vi "Add Item To Scene.vi"(8 "error in":errorcluster, 10 "Tree Element":T1, 11 "Scene In":refnum<vi>) -> (0 "error out":errorcluster, 3 "Scene Out":refnum<vi>)   [LabVIEW 2015]
doc: "This VI adds all the items to the scene"
uses:
  <vilib>/robotics/Kinematics/Plotting/Tree Element.ctl
  <vilib>/robotics/Kinematics/Plotting/Element Type.ctl
  <vilib>/robotics/Kinematics/Plotting/Joint Type.ctl
  <vilib>/picture/3D Picture Control/Object/Create Object (name).vi
  <vilib>/Utility/AngleManip/Degrees to Radians (Scalar DBL).vi
  <vilib>/picture/3D Picture Control/NI_3D Picture Control.lvlib
  <vilib>/Utility/AngleManip/NI_AngleManipulation.lvlib
  <vilib>/robotics/Kinematics/Plotting/NI_Robotics_3DKinematics.lvlib
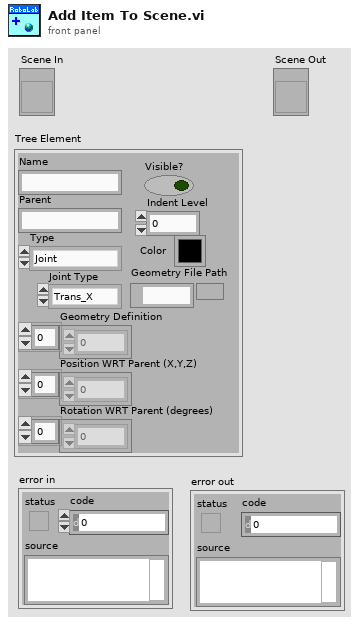
[diagram p1: front panel]
types:
  T1 = typedef "NI_Robotics_3DKinematics.lvlib/Tree Element.ctl" = cluster{"Name":string, "Parent":string, "Type":T2, "Visible?":bool, "Geometry Definition":dbl[], "Position WRT Parent (X,Y,Z)":dbl[], "Rotation WRT Parent (degrees)":dbl[], "Joint Type":T3, "Geometry File Path":path, "Indent Level":i32, "Color":u32}
  T2 = typedef "NI_Robotics_3DKinematics.lvlib/Element Type.ctl" = enum16{"Joint", "Box", "Cylinder", "Cone", "Sphere", "ASE File", "VRML File", "STL File", "Space"}
  T3 = typedef "NI_Robotics_3DKinematics.lvlib/Joint Type.ctl" = enum16{"Trans_X", "Trans_Y", "Trans_Z", "Rot_X", "Rot_Y", "Rot_Z", "None"}
  T4 = enum16{"Overall", "Per Primitive", "Per Vertex", "Binding Off"}
  T5 = cluster{"Position WRT Parent (X,Y,Z)[0]":dbl, "Position WRT Parent (X,Y,Z)[1]":dbl, "Position WRT Parent (X,Y,Z)[2]":dbl}
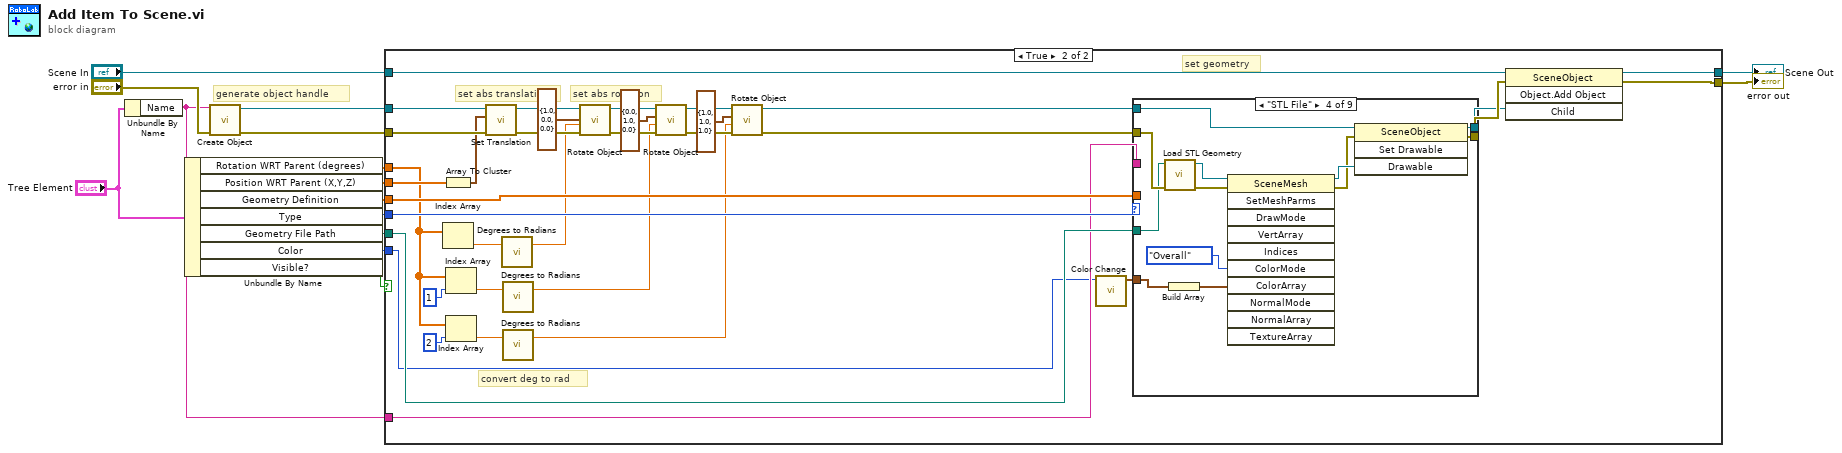
[diagram p0: block diagram]
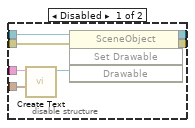
[diagram p4: hidden frame]
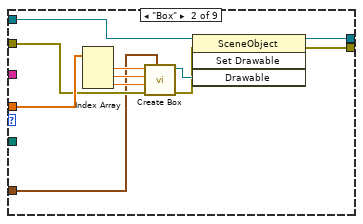
[diagram p5: hidden frame]
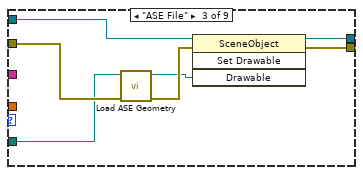
[diagram p6: hidden frame]
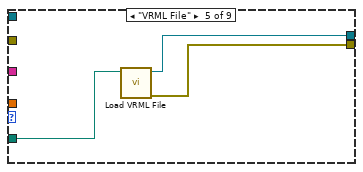
[diagram p7: hidden frame]
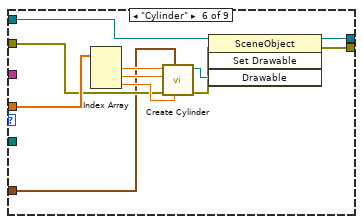
[diagram p8: hidden frame]
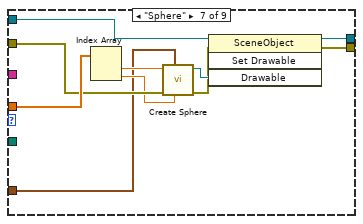
[diagram p9: hidden frame]
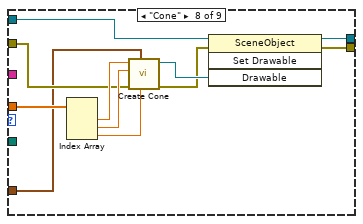
[diagram p10: hidden frame]
diagram:
  # "generate object handle"
  n1 = Unbundle By Name("Tree Element") -> ("Name"=w6:string)
  n2 = Unbundle By Name("Tree Element") -> ("Rotation WRT Parent (degrees)"=w4:dbl[], "Position WRT Parent (X,Y,Z)"=w12:dbl[], "Geometry Definition"=w10:dbl[], "Type"=w9:T2, "Geometry File Path"=w7:path, "Color"=w5:u32, "Visible?"=w1:bool)
  n3 = call-poly <vilib>:"Create Object.vi"("error in (no error)"="error in", "Name"=w6) -> ("error out"=w13:errorcluster, "Scene:New Object"=w14:refnum<vi>)  [unwired: 8 in]
  n4 = case shown="True" w1 {
    tunnel: w14 -> [_ w52]
    tunnel: w13 -> [w16 w51]
    tunnel: w12 -> [_ w50]
    tunnel: w10 -> [_ w48]
    tunnel: w9 -> [_ w46]
    tunnel: "Scene In" -> [w17 w45]
    tunnel: w7 -> [_ w44]
    tunnel: w6 -> [_ w43]
    tunnel: w5 -> [_ w32]
    tunnel: w4 -> [_ w20]
    tunnel: [w17 w19] -> w3
    tunnel: [w16 w18] -> w2
    frame False {
    }
    frame True {
      # "set abs rotation"
      # "set abs translation"
      # "set geometry"
      # "convert deg to rad"
      n5 = Array To Cluster(array=w50) -> (cluster=w39:T5)
      n6 = Index Array(array=w20) -> (element=w38:dbl)  [unwired: 1 in]
      n7 = Index Array(array=w20, index=1) -> (element=w31:dbl)
      n8 = Index Array(array=w20, index=2) -> (element=w23:dbl)
      n9 = call <vilib>:"Set Translation.vi"("error in (no error)"=w51, "Translation"=w39, "Scene Object"=w52) -> ("error out"=w41:errorcluster, "Translated Object"=w40:refnum<vi>)  [unwired: 7 out]
      n10 = call-poly <vilib>:"Degrees to Radians.vi"("angle (deg)"=w38) -> ("angle (rad)"=w37:dbl)  [unwired: 2 in]
      n11 = call-poly <vilib>:"Degrees to Radians.vi"("angle (deg)"=w31) -> ("angle (rad)"=w29:dbl)  [unwired: 2 in]
      n12 = call-poly <vilib>:"Degrees to Radians.vi"("angle (deg)"=w23) -> ("angle (rad)"=w24:dbl)  [unwired: 2 in]
      n13 = call <vilib>:"Rotate Object.vi"("error in (no error)"=w41, "Angle"=w37, "Axis"=cluster{"X":sgl, "Y":sgl, "Z":sgl} {"X"=1.0, "Y"=0.0, "Z"=0.0}, "Scene.Object In"=w40) -> ("error out"=w34:errorcluster, "Scene.Object Out"=w35:refnum<vi>)  [unwired: 6 in]
      n14 = call <vilib>:"Rotate Object.vi"("error in (no error)"=w34, "Angle"=w29, "Axis"=cluster{"X":sgl, "Y":sgl, "Z":sgl} {"X"=0.0, "Y"=1.0, "Z"=0.0}, "Scene.Object In"=w35) -> ("error out"=w27:errorcluster, "Scene.Object Out"=w28:refnum<vi>)  [unwired: 6 in]
      n15 = call <vilib>:"Rotate Object.vi"("error in (no error)"=w27, "Angle"=w24, "Axis"=cluster{"X":sgl, "Y":sgl, "Z":sgl} {"X"=1.0, "Y"=1.0, "Z"=1.0}, "Scene.Object In"=w28) -> ("error out"=w21:errorcluster, "Scene.Object Out"=w22:refnum<vi>)  [unwired: 6 in]
      n16 = call <vilib>:"Color Change.vi"("Color"=w32) -> ("RGBA"=w42:cluster{"R":sgl, "G":sgl, "B":sgl, "A":sgl})  [unwired: 1 in, 9 out]
      n17 = case shown="\"STL File\"" w46 {
        tunnel: w22 -> [w56 w78 w79 w97 _ w111 w121 w132 w134]
        tunnel: [w55 w77 w85 w96 w99 w110 w120 w131 w134] -> w47
        tunnel: w48 -> [_ w76 _ _ _ w109 w119 w130 _]
        tunnel: w21 -> [w58 w71 w84 w95 _ w104 w117 w123 w133]
        tunnel: [w54 w69 w82 w94 w98 w102 w115 w125 w133] -> w49
        tunnel: w44 -> [_ _ w81 w93 w100 _ _ _ _]
        tunnel: w43 -> [w57 _ _ _ _ _ _ _ _]
        tunnel: w42 -> [w53 w68 _ w92 _ w101 w112 w122 _]
        frame "Joint", Default {
          n18 = disable-structure shown="Enabled" {
            disable-tunnel: w58 -> [w64 w66]
            disable-tunnel: w57 -> [w63 _]
            disable-tunnel: w56 -> [w62 w67]
            disable-tunnel: [w61 w67] -> w55
            disable-tunnel: [w60 w66] -> w54
            disable-tunnel: w53 -> [w59 _]
            frame Disabled {
              n19 = call <vilib>:"Create Text.vi"("Color"=w59, "Text"=w63) -> ("New Text Refnum"=w65:refnum<vi>)  [unwired: 2 in, 7 out]
              n20 = invoke class="SceneObject" method="Set Drawable"(reference=w62, error in=w64, "Drawable"=w65) -> (reference out=w61:refnum<vi>, error out=w60:errorcluster)  [unwired: 1 in, 2 out]
            }
            frame Enabled {
            }
          }
        }
        frame "Box" {
          n21 = Index Array(array=w76) -> (element #1=w75:dbl, element #2=w74:dbl, element #3=w73:dbl)  [unwired: 3 in]
          n22 = call <vilib>:"Create Box.vi"("Color"=w68, "error in (no error)"=w71, "Length Z"=w73, "Length Y"=w74, "Length X"=w75) -> ("error out"=w70:errorcluster, "New Box Refnum"=w72:refnum<vi>)  [unwired: 5 out]
          n23 = invoke class="SceneObject" method="Set Drawable"(reference=w78, error in=w70, "Drawable"=w72) -> (reference out=w77:refnum<vi>, error out=w69:errorcluster)  [unwired: 1 in, 2 out]
        }
        frame "ASE File" {
          n24 = call <vilib>:"Load ASE Geometry.vi"("error in (no error)"=w84, "Model File"=w81) -> ("error out"=w83:errorcluster, "New Mesh Refnum"=w80:refnum<vi>)  [unwired: 2 in, 6 out]
          n25 = invoke class="SceneObject" method="Set Drawable"(reference=w79, error in=w83, "Drawable"=w80) -> (reference out=w85:refnum<vi>, error out=w82:errorcluster)  [unwired: 1 in, 2 out]
        }
        frame "STL File" {
          n26 = call <vilib>:"Load STL Geometry.vi"("error in (no error)"=w95, "Model File"=w93) -> ("error out"=w87:errorcluster, "New Mesh Refnum"=w91:refnum<vi>)  [unwired: 8 out]
          n27 = Build Array(w92) -> (w88:cluster{"R":sgl, "G":sgl, "B":sgl, "A":sgl}[])
          n28 = invoke class="SceneMesh" method="SetMeshParms"(reference=w91, error in=w87, "ColorMode"=T4."Overall" ("Color Binding Mode"), "ColorArray"=w88) -> (reference out=w90:refnum<vi>, error out=w86:errorcluster)  [unwired: 7 in, 9 out]
          n29 = invoke class="SceneObject" method="Set Drawable"(reference=w97, error in=w86, "Drawable"=w90) -> (reference out=w96:refnum<vi>, error out=w94:errorcluster)  [unwired: 1 in, 2 out]
        }
        frame "VRML File" {
          n30 = call <vilib>:"Load VRML File.vi"("Path"=w100) -> ("error out"=w98:errorcluster, "Scene:Read Scene File"=w99:refnum<vi>)  [unwired: 1 in, 8 out]
        }
        frame "Cylinder" {
          n31 = Index Array(array=w109) -> (element #1=w108:dbl, element #2=w107:dbl, element #3=w106:dbl)  [unwired: 3 in]
          n32 = call <vilib>:"Create Cylinder.vi"("Detail"=w106, "Color"=w101, "error in (no error)"=w104, "Radius"=w107, "Height"=w108) -> ("error out"=w103:errorcluster, "New Cylinder Refnum"=w105:refnum<vi>)  [unwired: 5 out]
          n33 = invoke class="SceneObject" method="Set Drawable"(reference=w111, error in=w103, "Drawable"=w105) -> (reference out=w110:refnum<vi>, error out=w102:errorcluster)  [unwired: 1 in, 2 out]
        }
        frame "Sphere" {
          n34 = Index Array(array=w119) -> (element #1=w114:dbl, element #2=w113:dbl)  [unwired: 2 in]
          n35 = call <vilib>:"Create Sphere.vi"("Detail"=w113, "Color"=w112, "error in (no error)"=w117, "Radius"=w114) -> ("error out"=w116:errorcluster, "New Sphere Refnum"=w118:refnum<vi>)  [unwired: 1 in, 5 out]
          n36 = invoke class="SceneObject" method="Set Drawable"(reference=w121, error in=w116, "Drawable"=w118) -> (reference out=w120:refnum<vi>, error out=w115:errorcluster)  [unwired: 1 in, 2 out]
        }
        frame "Cone" {
          n37 = Index Array(array=w130) -> (element #1=w129:dbl, element #2=w128:dbl, element #3=w127:dbl)  [unwired: 3 in]
          n38 = call <vilib>:"Create Cone.vi"("Detail"=w127, "Color"=w122, "error in (no error)"=w123, "Radius"=w128, "Height"=w129) -> ("error out"=w124:errorcluster, "New Cone Refnum"=w126:refnum<vi>)  [unwired: 5 out]
          n39 = invoke class="SceneObject" method="Set Drawable"(reference=w132, error in=w124, "Drawable"=w126) -> (reference out=w131:refnum<vi>, error out=w125:errorcluster)  [unwired: 1 in, 2 out]
        }
        frame "Space" {
        }
      }
      n40 = invoke class="SceneObject" method="Object.Add Object"(reference=w45, error in=w49, "Child"=w47) -> (reference out=w19:refnum<vi>, error out=w18:errorcluster)  [unwired: 1 in, 2 out]
    }
  }
  "error out" <- w2
  "Scene Out" <- w3
